vi "user interface.vi"() -> ()   [LabVIEW 2018]
uses:
  <vilib>/Tufts CEEO ROS for LabVIEW Software/ROS/Code/SubVIs/_ROSControl.ctl
  <vilib>/Tufts CEEO ROS for LabVIEW Software/ROS/Code/SubVIs/_ROSDirection.ctl
  <vilib>/Tufts CEEO ROS for LabVIEW Software/ROS/Code/Console/Servers/ServerSubs/TopicDef.ctl
  <vilib>/Tufts CEEO ROS for LabVIEW Software/ROS/MessageBuilding/std_msgs/subs/stringScalar.vi
panel:
  in  "X POSITION":dbl
  out "ROBOT SPEED":dbl(knob) scale=0.0..10.0
  in  "Update Time (ms)":u32=300
  out "XY Graph":cluster{"Y":dbl[], "Y":dbl[]}[](graph)
  out "Robot state":string
  in  "stop":bool
  in  "Start Scanning":bool
  in  "Start Registring the Robot Position":bool
  out "Scan Details":T1={"Min. Angle (rad)"=-2.3561899662017822, "Max. Angle (rad)"=2.3561899662017822, "Angle Incr. (rad)"=0.006554075051099062, "Time Inc. (s)"=0.0, "Scan Time (s)"=0.0, "Min. Range (m)"=0.10000000149011612, "Max. Range (m)"=1.0089348943138683e-42}
  out "Laser Scan Plot (in Husky Frame)":cluster{dbl[], dbl[]}(graph)
  out "Odom Error Out":errorcluster
  out "Scan Error Out":errorcluster
  out "Husky EKF Odometry":T2={"PoseCovariance"={"Pose"={"Position\n(xyz)"={"x"=2.1588546690121686, "y"=0.6824320147682317, "z"=0.0}, "Orientation\n(Quaternions)"={"x"=0.0, "y"=0.0, "z"=-0.6154075833582808, "w"=0.7882090499005455}}, "Covariance[1,1]"=150.49515067805697}}
  out "2D Pose":cluster{"x":dbl, "y":dbl}={"x"=2.1588546690121686, "y"=0.6824320147682317}
  in  "Manual Mode":bool
  out "ROS out":T3={"topic port"=0, "Node"="", "topic"="", "type"="", "node port"=0, "error "={"status"=FALSE, "code"=0, "source"=""}, "Direction"=enum."Node", "Update (ms)"=1, "FIFO size"=1}
  in  "DOWN":bool
  in  "TOP":bool
  in  "RIGHT":bool
  in  "LEFT":bool
  in  "THETA POSITION":dbl
  out "error out":errorcluster
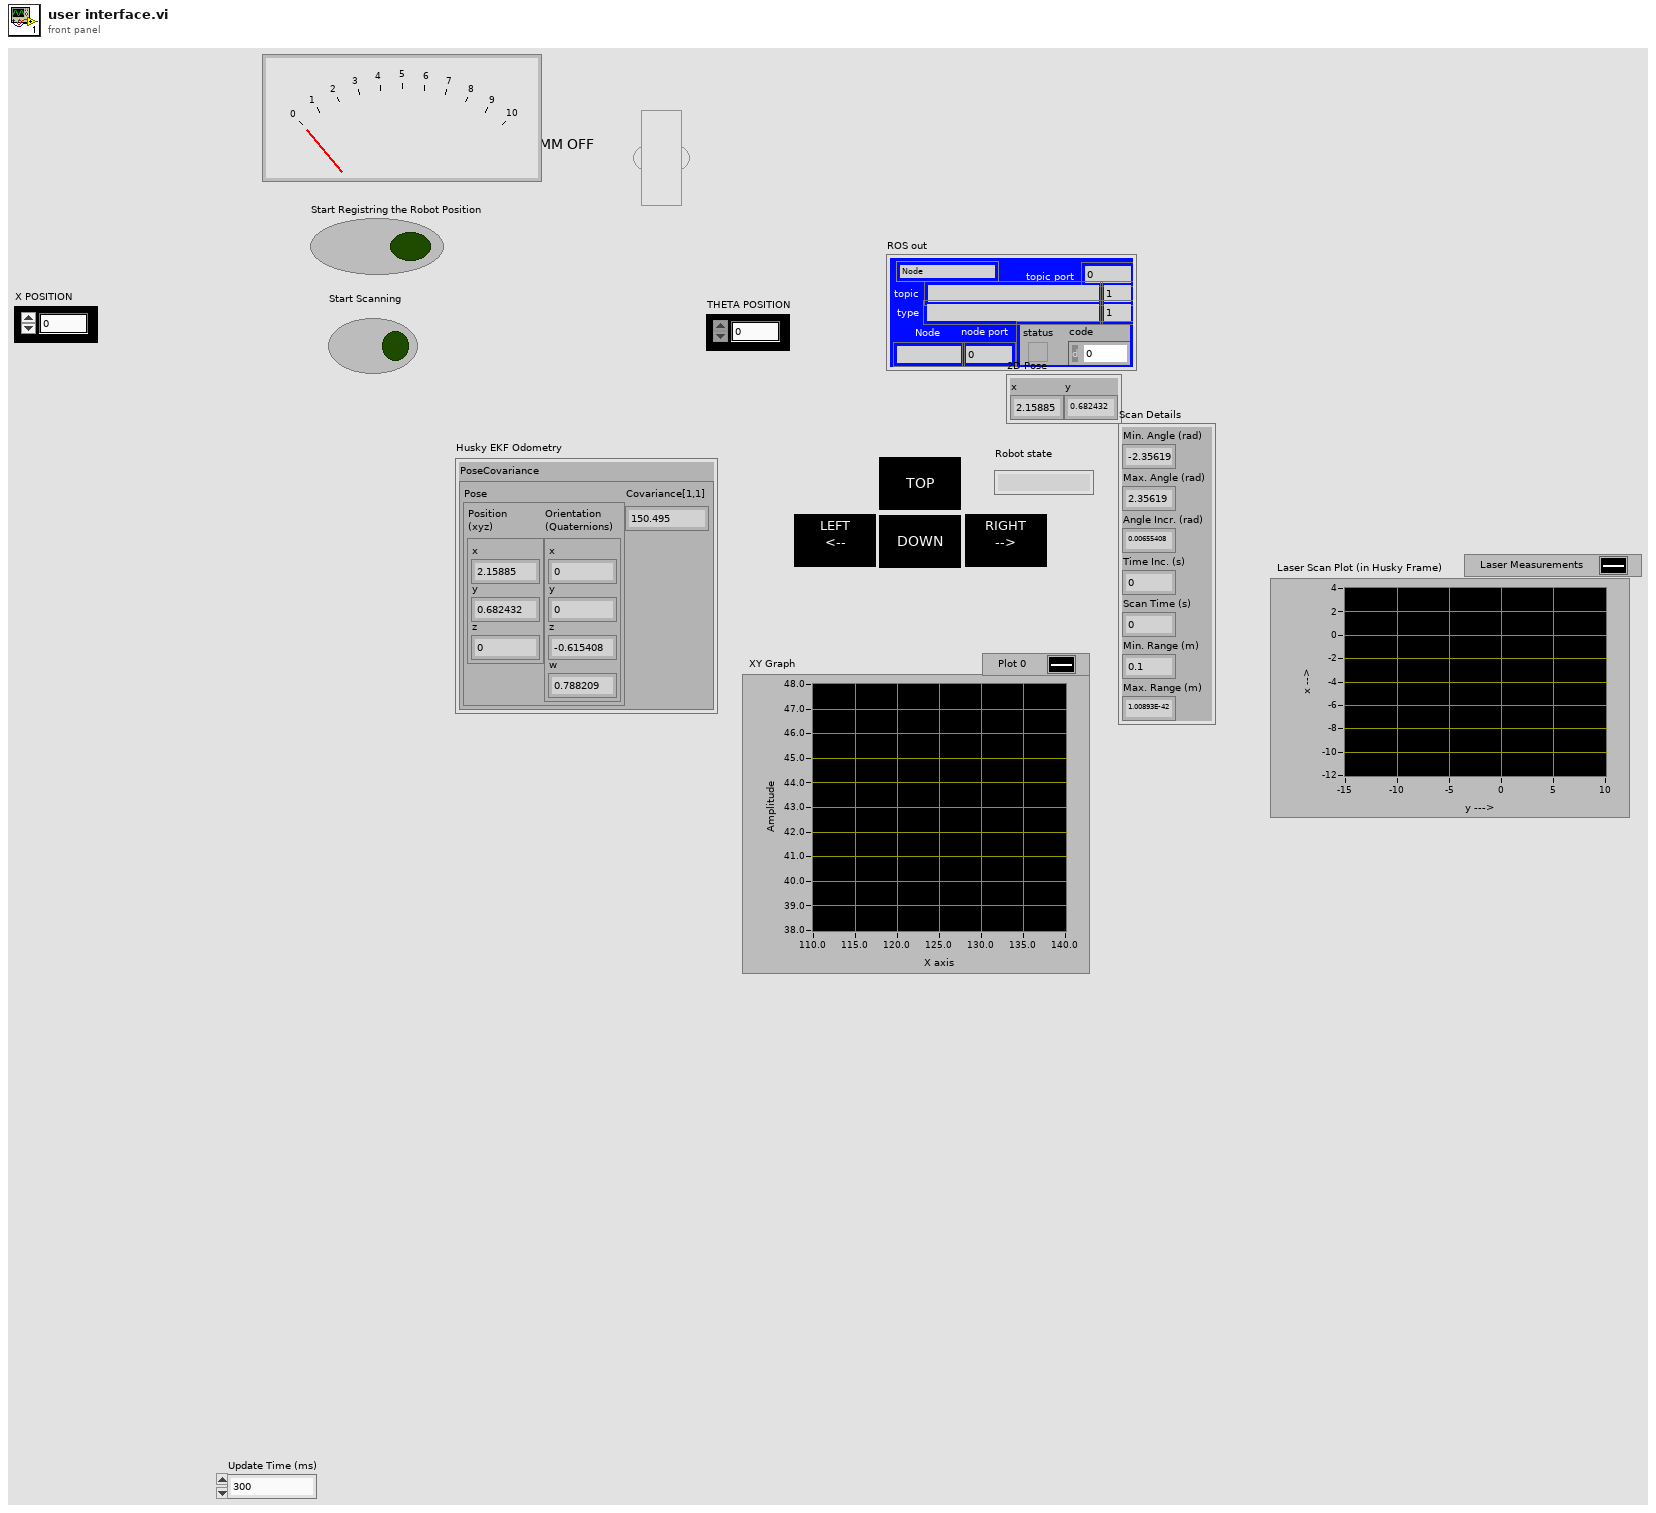
[diagram p1: front panel]
types:
  T1 = cluster{"Min. Angle (rad)":dbl, "Max. Angle (rad)":dbl, "Angle Incr. (rad)":dbl, "Time Inc. (s)":dbl, "Scan Time (s)":dbl, "Min. Range (m)":dbl, "Max. Range (m)":dbl}
  T2 = cluster{"PoseCovariance":cluster{"Pose":cluster{"Position\n(xyz)":cluster{"x":dbl, "y":dbl, "z":dbl}, "Orientation\n(Quaternions)":cluster{"x":dbl, "y":dbl, "z":dbl, "w":dbl}}, "Covariance[1,1]":dbl}}
  T3 = typedef "_ROSControl.ctl" = cluster{"topic port":u16, "Node":string, "topic":string, "type":string, "node port":u16, "error ":errorcluster, "Direction":T4, "Update (ms)":u16, "FIFO size":u16}
  T4 = typedef "_ROSDirection.ctl" = enum16{"Node", "Publisher", "Subscriber", "ServiceClient", "ServiceProvider"}
  T5 = typedef "TopicDef.ctl" = cluster{"Topic":string, "Type":string, "Action":T4, "Update (ms)":u16, "queue size":u16}
  T6 = cluster{"PoseCovariance":cluster{"Pose":cluster{"Point":cluster{"x":dbl, "y":dbl, "z":dbl}, "Quaternion":cluster{"x":dbl, "y":dbl, "z":dbl, "w":dbl}}, "Covariance":dbl}}
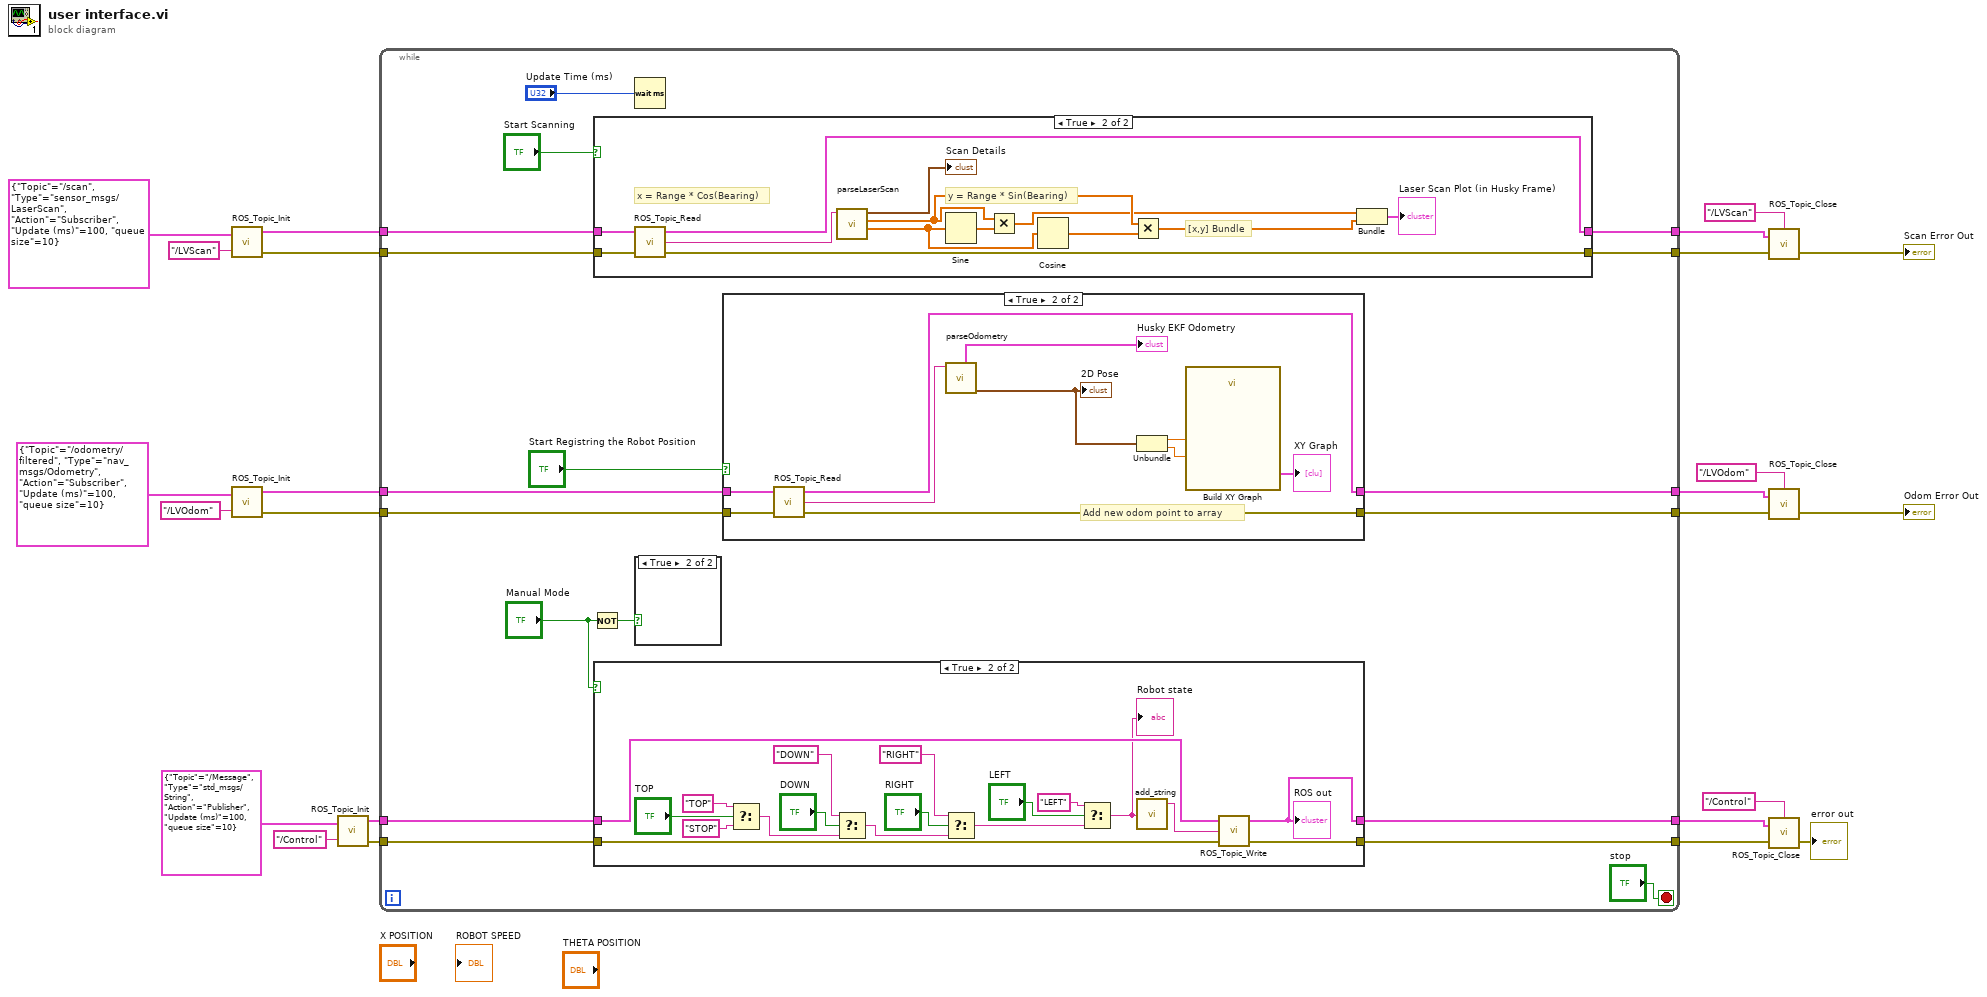
[diagram p0: block diagram]
diagram:
  n1 = call <vilib>:"ROS_Topic_Init.vi"("Definitions"=T5 {"Topic"="/scan", "Type"="sensor_msgs/LaserScan", "Action"=enum."Subscriber", "Update (ms)"=100, "queue size"=10}, "node"="/LVScan") -> ("ROS out"=w11:T3, "error out"=w10:errorcluster)  [unwired: 1 in]
  n2 = call <vilib>:"ROS_Topic_Init.vi"("Definitions"=T5 {"Topic"="/odometry/filtered", "Type"="nav_msgs/Odometry", "Action"=enum."Subscriber", "Update (ms)"=100, "queue size"=10}, "node"="/LVOdom") -> ("ROS out"=w15:T3, "error out"=w14:errorcluster)  [unwired: 1 in]
  n3 = call <vilib>:"ROS_Topic_Init.vi"("Definitions"=T5 {"Topic"="/Message", "Type"="std_msgs/String", "Action"=enum."Publisher", "Update (ms)"=100, "queue size"=10}, "node"="/Control") -> ("ROS out"=w19:T3, "error out"=w18:errorcluster)  [unwired: 1 in]
  n4 = while {
    tunnel: [w29] -> w24
    tunnel: w19 -> [w39]
    tunnel: w18 -> [w38]
    tunnel: w15 -> [w37]
    tunnel: w14 -> [w36]
    tunnel: w11 -> [w35]
    tunnel: w10 -> [w34]
    tunnel: [w33] -> w8
    tunnel: [w32] -> w7
    tunnel: [w31] -> w4
    tunnel: [w30] -> w3
    tunnel: [w28] -> w1
    stop <- "stop" stop-if-true
    n5 = Not(x="Manual Mode") -> (.not. x?=w26:bool)
    n6 = case shown="True" "Start Scanning" {
      tunnel: [w44 w57] -> w32
      tunnel: [w43 w56] -> w33
      tunnel: w35 -> [w44 w55]
      tunnel: w34 -> [w43 w54]
      frame False {
      }
      frame True {
        # "[x,y] Bundle"
        # "y = Range * Sin(Bearing)"
        # "x = Range * Cos(Bearing)"
        n7 = call <vilib>:"ROS_Topic_Read.vi"("error in (no error)"=w54, "ROS in"=w55) -> ("error out"=w56:errorcluster, "Reply"=w53:string, "ROS out"=w57:T3)  [unwired: 1 in]
        n8 = call "parseLaserScan.vi"("msg in"=w53) -> ("Bearing Array"=w51:dbl[], "Range Array"=w50:sgl[], "Scan Details"=→"Scan Details":T1)  [unwired: 3 in, 1 out]
        n9 = Sine(x=w51) -> (sin(x)=w49:dbl[])
        n10 = Multiply(x=w50, y=w49) -> (x*y=w46:dbl[])
        n11 = Cosine(x=w51) -> (cos(x)=w52:dbl[])
        n12 = Multiply(x=w50, y=w52) -> (x*y=w47:dbl[])
        n13 = Bundle(w46, w47) -> (→"Laser Scan Plot (in Husky Frame)":cluster{dbl[], dbl[]})  [unwired: 1 in]
      }
    }
    n14 = case shown="True" "Manual Mode" {
      tunnel: w38 -> [w70 w86]
      tunnel: w39 -> [w71 w87]
      tunnel: [w71 w88] -> w29
      tunnel: [w70 w89] -> w28
      frame False {
      }
      frame True {
        n15 = Select(t="TOP", s="TOP", f="STOP") -> (s? t:f=w85:string)
        n16 = Select(t="DOWN", s="DOWN", f=w85) -> (s? t:f=w84:string)
        n17 = Select(t="RIGHT", s="RIGHT", f=w84) -> (s? t:f=w76:string)
        n18 = Select(t="LEFT", s="LEFT", f=w76) -> (s? t:f=w73:string)
        "Robot state" <- w73
        n19 = call-poly <vilib>:"add_string.vi"("String"=w73) -> ("msg out"=w72:string)  [unwired: 4 in]
        n20 = call <vilib>:"ROS_Topic_Write.vi"("error in (no error)"=w86, "Msg in"=w72, "ROS in"=w87) -> ("error out"=w89:errorcluster, "ROS out"=w88:T3)  [unwired: 1 in]
        "ROS out" <- w88
      }
    }
    n21 = Wait (ms)(milliseconds to wait="Update Time (ms)") -> ()  [unwired: 1 out]
    n22 = case shown="True" w26 {
      frame False {
      }
      frame True {
      }
    }
    n23 = case shown="True" "Start Registring the Robot Position" {
      tunnel: w37 -> [w59 w69]
      tunnel: w36 -> [w58 w68]
      tunnel: [w59 w67] -> w30
      tunnel: [w58 w66] -> w31
      frame False {
      }
      frame True {
        # "Add new odom point to array"
        n24 = call <vilib>:"ROS_Topic_Read.vi"("error in (no error)"=w68, "ROS in"=w69) -> ("error out"=w66:errorcluster, "Reply"=w65:string, "ROS out"=w67:T3)  [unwired: 1 in]
        n25 = call "parseOdometry.vi"("msg in"=w65) -> ("Odometry"=→"Husky EKF Odometry":T6, "Pose 2D"=w63:cluster{"x":dbl, "y":dbl})  [unwired: 3 in, 3 out]
        "2D Pose" <- w63
        n26 = Unbundle(w63) -> ("x"=w61:dbl, "y"=w60:dbl)
        n27 = call "Build XY Graph"("Y Input"=w60, "X Input"=w61) -> ("XY Graph"=→"XY Graph":cluster{"X":dbl[], "Y":dbl[]}[])  [unwired: 8 in, 1 out]
      }
    }
  }
  n28 = call <vilib>:"ROS_Topic_Close.vi"("error in"=w8, "ROS in"=w7, "node"="/LVScan") -> ("error out"=→"Scan Error Out":errorcluster)  [unwired: 1 in]
  n29 = call <vilib>:"ROS_Topic_Close.vi"("error in"=w4, "ROS in"=w3, "node"="/LVOdom") -> ("error out"=→"Odom Error Out":errorcluster)  [unwired: 1 in]
  n30 = call <vilib>:"ROS_Topic_Close.vi"("error in"=w1, "ROS in"=w24, "node"="/Control") -> ("error out"=→"error out":errorcluster)  [unwired: 1 in]
